vi "gl_Volume Entry UI globals.vi"() -> ()   [LabVIEW 2017]
uses:
  Typedefs/Volume entry ctrl refs cluster.ctl
panel:
  in  "Volume entry ctrl refs":T1
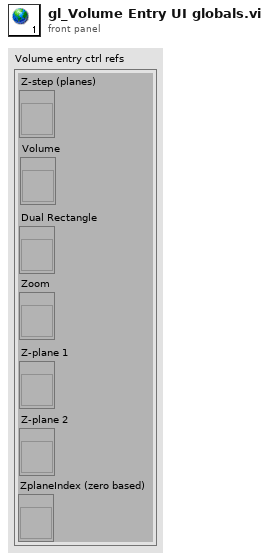
[diagram p1: front panel]
types:
  T1 = typedef "Volume entry ctrl refs cluster.ctl" = cluster{"Z-step (planes)":refnum<vi>, "Volume":refnum<vi>, "Dual Rectangle":refnum<vi>, "Zoom":refnum<vi>, "Z-plane 1":refnum<vi>, "Z-plane 2":refnum<vi>, "ZplaneIndex (zero based)":refnum<vi>}
diagram:
